vi "KGN Get actual Values.vi"(7 "scaling":dbl, 8 "Fehler (Eingang, kein Fehler)":errorcluster, 9 "Info Cluster":T1, 10 "VISA-Referenz (Eingang)":refnum<visa-resource-name>, 11 "device (Eingang)":u32) -> (0 "Fehler (Ausgang)":errorcluster, 1 "Info Cluster out":T1, 2 "VISA-Referenz (Ausgang)":refnum<visa-resource-name>, 3 "dup device (Ausgang)":u32, 4 "actual Values Cluster":T6 {"Cluster"."PumpModeGeneral-Cluster"."dry mode" items=["wet", "dry"]; "Cluster"."PumpModeGeneral-Cluster"."control mode" items=["static", "pid"]; "Cluster"."PumpMode-Cluster"."concentratio mode" items=["water", "reagent"]; "Cluster"."PumpMode-Cluster"."Reagent" items=["HCl", "HF", "NH3", "HG", "PPM", "ORGANIC"]}, 5 "Kommandos gesendet":string, 6 "connected":bool)   [LabVIEW 2020, in "Linearisierung v2.lvlib" / "Gasteiler.lvlib" / "HovaCAL_Interface.lvlib" / "KGN.lvlib" / "KGN GUI Get.lvlib"]
uses:
  KGN GUI Get.lvlib
  Controls/Info Cluster.ctl
  Controls/Pump Dry Mode.ctl
  Controls/Pump Control Mode.ctl
  Controls/Pump Concentration Mode.ctl
  Controls/Reagent.ctl
  Controls/Controls.lvlib
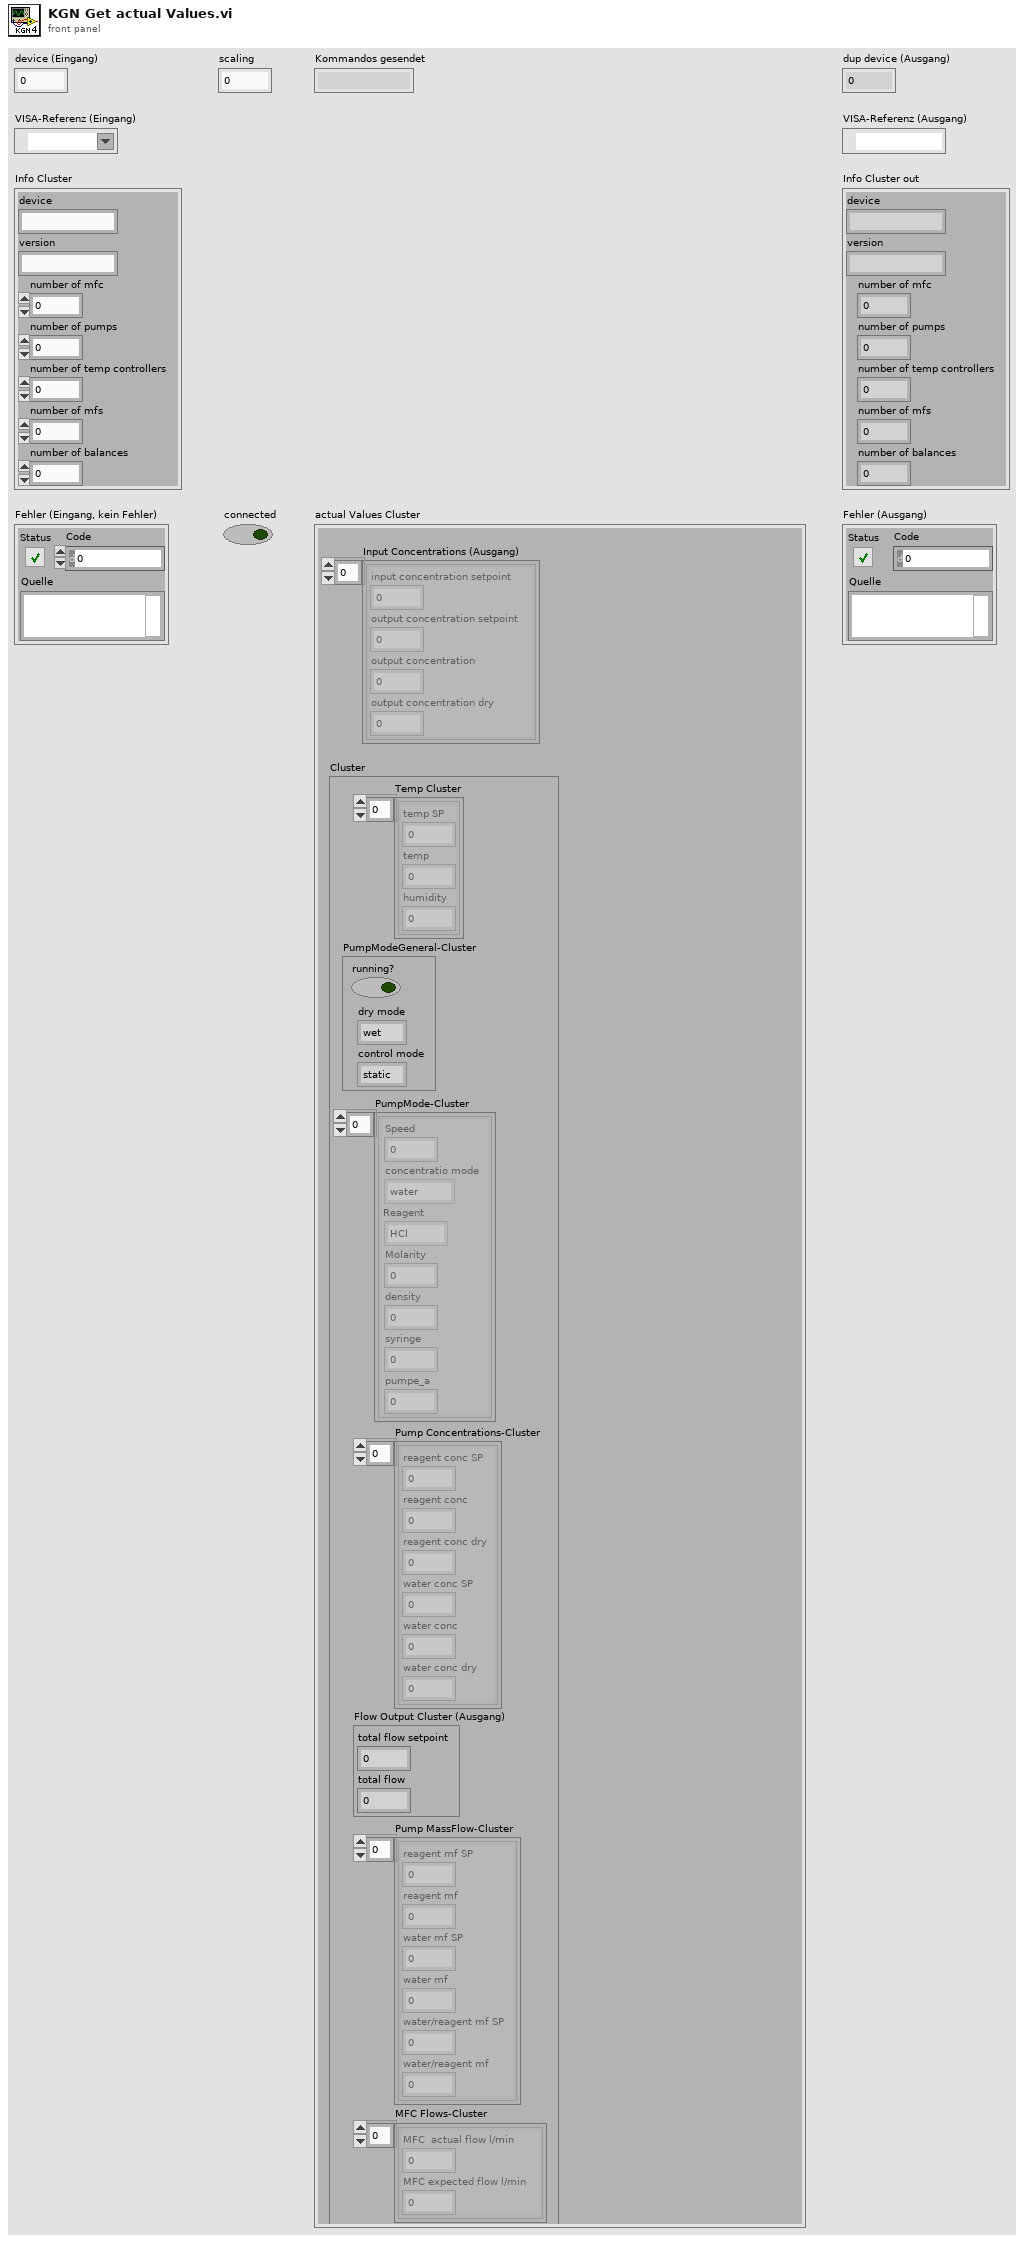
[diagram p1: front panel]
types:
  T1 = typedef "Linearisierung v2.lvlib/Gasteiler.lvlib/HovaCAL_Interface.lvlib/Controls.lvlib/Info Cluster.ctl" = cluster{"device":string, "version":string, "number of mfc":i32, "number of pumps":i32, "number of temp controllers":i32, "number of mfs":i32, "number of balances":i32}
  T2 = typedef "Linearisierung v2.lvlib/Gasteiler.lvlib/HovaCAL_Interface.lvlib/Controls.lvlib/Pump Dry Mode.ctl" = i32
  T3 = typedef "Linearisierung v2.lvlib/Gasteiler.lvlib/HovaCAL_Interface.lvlib/Controls.lvlib/Pump Control Mode.ctl" = u32
  T4 = typedef "Linearisierung v2.lvlib/Gasteiler.lvlib/HovaCAL_Interface.lvlib/Controls.lvlib/Pump Concentration Mode.ctl" = i32
  T5 = typedef "Linearisierung v2.lvlib/Gasteiler.lvlib/HovaCAL_Interface.lvlib/Controls.lvlib/Reagent.ctl" = i32
  T6 = cluster{"Input Concentrations (Ausgang)":cluster{"input concentration setpoint":dbl, "output concentration setpoint":dbl, "output concentration":dbl, "output concentration dry":dbl}[], "Cluster":cluster{"Temp Cluster":cluster{"temp SP":dbl, "temp":dbl, "humidity":dbl}[], "PumpModeGeneral-Cluster":cluster{"running?":bool, "dry mode":T2, "control mode":T3}, "PumpMode-Cluster":cluster{"Speed":dbl, "concentratio mode":T4, "Reagent":T5, "Molarity":dbl, "density":dbl, "syringe":dbl, "pumpe_a":dbl}[], "Pump Concentrations-Cluster":cluster{"reagent conc SP":dbl, "reagent conc":dbl, "reagent conc dry":dbl, "water conc SP":dbl, "water conc":dbl, "water conc dry":dbl}[], "Flow Output Cluster (Ausgang)":cluster{"total flow setpoint":dbl, "total flow":dbl}, "Pump MassFlow-Cluster":cluster{"reagent mf SP":dbl, "reagent mf":dbl, "water mf SP":dbl, "water mf":dbl, "water/reagent mf SP":dbl, "water/reagent mf":dbl}[], "MFC Flows-Cluster":cluster{"MFC  actual flow l/min":dbl, "MFC expected flow l/min":dbl}[]}}
  T7 = cluster{"input concentration setpoint":dbl, "output concentration setpoint":dbl, "output concentration":dbl, "output concentration dry":dbl}[]
  T8 = cluster{"temp SP":dbl, "temp":dbl, "humidity":dbl}[]
  T9 = cluster{"running?":bool, "dry mode":T2, "control mode":T3}
  T10 = cluster{"Speed":dbl, "concentratio mode":T4, "Reagent":T5, "Molarity":dbl, "density":dbl, "syringe":dbl, "pump_a":dbl}[]
  T11 = cluster{"reagent conc SP":dbl, "reagent conc":dbl, "reagent conc dry":dbl, "water conc SP":dbl, "water conc":dbl, "water conc dry":dbl}[]
  T12 = cluster{"reagent mf SP":dbl, "reagent mf":dbl, "water mf SP":dbl, "water mf":dbl, "water/reagent mf SP":dbl, "water/reagent mf":dbl}[]
  T13 = cluster{"total flow setpoint":dbl, "total flow":dbl}
  T14 = cluster{"MFC  actual flow l/min":dbl, "MFC expected flow l/min":dbl}[]
  T15 = cluster{"Temp Cluster":cluster{"temp SP":dbl, "temp":dbl, "humidity":dbl}[], "PumpModeGeneral-Cluster":cluster{"running?":bool, "dry mode":T2, "control mode":T3}, "PumpMode-Cluster":cluster{"Speed":dbl, "concentratio mode":T4, "Reagent":T5, "Molarity":dbl, "density":dbl, "syringe":dbl, "pump_a":dbl}[], "Pump Concentrations-Cluster":cluster{"reagent conc SP":dbl, "reagent conc":dbl, "reagent conc dry":dbl, "water conc SP":dbl, "water conc":dbl, "water conc dry":dbl}[], "Flow Output Cluster (Ausgang)":cluster{"total flow setpoint":dbl, "total flow":dbl}, "Pump MassFlow-Cluster":cluster{"reagent mf SP":dbl, "reagent mf":dbl, "water mf SP":dbl, "water mf":dbl, "water/reagent mf SP":dbl, "water/reagent mf":dbl}[], "MFC Flows (Ausgang)":cluster{"MFC  actual flow l/min":dbl, "MFC expected flow l/min":dbl}[]}
  T16 = cluster{"Input Concentrations (Ausgang)":cluster{"input concentration setpoint":dbl, "output concentration setpoint":dbl, "output concentration":dbl, "output concentration dry":dbl}[], cluster{"Temp Cluster":cluster{"temp SP":dbl, "temp":dbl, "humidity":dbl}[], "PumpModeGeneral-Cluster":cluster{"running?":bool, "dry mode":T2, "control mode":T3}, "PumpMode-Cluster":cluster{"Speed":dbl, "concentratio mode":T4, "Reagent":T5, "Molarity":dbl, "density":dbl, "syringe":dbl, "pump_a":dbl}[], "Pump Concentrations-Cluster":cluster{"reagent conc SP":dbl, "reagent conc":dbl, "reagent conc dry":dbl, "water conc SP":dbl, "water conc":dbl, "water conc dry":dbl}[], "Flow Output Cluster (Ausgang)":cluster{"total flow setpoint":dbl, "total flow":dbl}, "Pump MassFlow-Cluster":cluster{"reagent mf SP":dbl, "reagent mf":dbl, "water mf SP":dbl, "water mf":dbl, "water/reagent mf SP":dbl, "water/reagent mf":dbl}[], "MFC Flows (Ausgang)":cluster{"MFC  actual flow l/min":dbl, "MFC expected flow l/min":dbl}[]}}
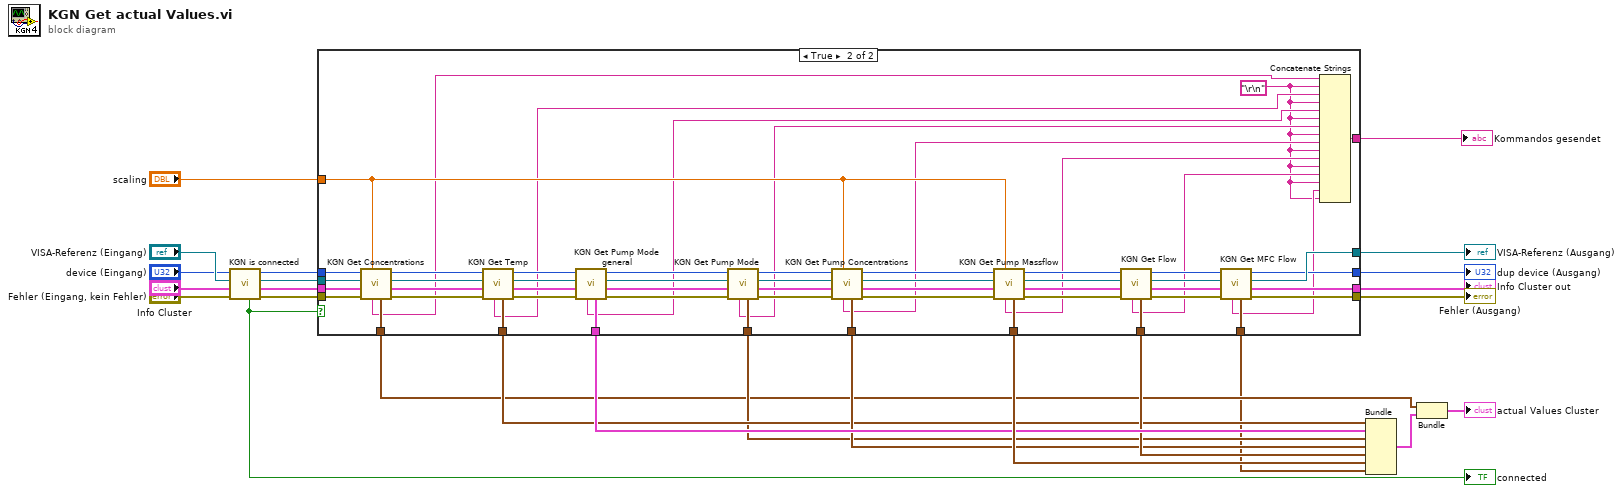
[diagram p0: block diagram]
diagram:
  n1 = call "KGN is connected.vi"("VISA-Ressourcenname"="VISA-Referenz (Eingang)", "device"="device (Eingang)") -> ("VISA-Ressourcenname out"=w22:refnum<visa-resource-name>, "dup device out"=w21:u32, "Boolesch"=w20:bool)  [unwired: 6 in, 1 out]
  "connected" <- w20
  n2 = case shown="True" w20 {
    tunnel: "Fehler (Eingang, kein Fehler)" -> [w27 w82]
    tunnel: [w27 w39] -> w8
    tunnel: w21 -> [w26 w81]
    tunnel: [_ w66] -> w6
    tunnel: "Info Cluster" -> [w24 w68]
    tunnel: [w26 w43] -> w9
    tunnel: "scaling" -> [_ w50]
    tunnel: [_ w57] -> w11
    tunnel: [_ w63] -> w12
    tunnel: [_ w54] -> w13
    tunnel: [_ w49] -> w14
    tunnel: [_ w60] -> w15
    tunnel: [_ w53] -> w18
    tunnel: w22 -> [w25 w67]
    tunnel: [w25 w45] -> w23
    tunnel: [w24 w41] -> w3
    tunnel: [_ w38] -> w2
    tunnel: [_ w28] -> w1
    frame False {
    }
    frame True {
      w29 = "\r\n"
      n3 = call "KGN Get Concentrations.vi"("scaling"=w50, "Fehler (Eingang, kein Fehler)"=w82, "Info Cluster"=w68, "VISA-Ressourcenname"=w67, "device (Eingang)"=w81) -> ("Fehler (Ausgang)"=w80:errorcluster, "Info Cluster out"=w65:T1, "VISA-Ressourcenname out"=w64:refnum<visa-resource-name>, "dup device (Ausgang)"=w79:u32, "Input Concentrations (Ausgang)"=w66:T7, "Kommandos gesendet"=w37:string)  [unwired: 1 in]
      n4 = call "KGN Get Temp.vi"("Fehler (Eingang, kein Fehler)"=w80, "Info Cluster"=w65, "VISA-Ressourcenname"=w64, "device (Eingang)"=w79) -> ("Fehler (Ausgang)"=w76:errorcluster, "Info Cluster out"=w61:T1, "VISA-Ressourcenname out"=w62:refnum<visa-resource-name>, "dup device (Ausgang)"=w74:u32, "Temp Cluster"=w63:T8, "Kommandos gesendet"=w36:string)  [unwired: 2 in]
      n5 = call "KGN Get Pump Mode general.vi"("Fehler (Eingang, kein Fehler)"=w76, "Info Cluster"=w61, "VISA-Ressourcenname"=w62, "device (Eingang)"=w74) -> ("Fehler (Ausgang)"=w75:errorcluster, "Info Cluster out"=w59:T1, "VISA-Ressourcenname out"=w58:refnum<visa-resource-name>, "dup device (Ausgang)"=w73:u32, "PumpModeGeneral-Cluster"=w60:T9, "Kommandos gesendet"=w35:string)  [unwired: 2 in]
      n6 = call "KGN Get Pump Mode.vi"("Fehler (Eingang, kein Fehler)"=w75, "Info Cluster"=w59, "VISA-Ressourcenname"=w58, "device (Eingang)"=w73) -> ("Fehler (Ausgang)"=w77:errorcluster, "Info Cluster out"=w56:T1, "VISA-Ressourcenname out"=w55:refnum<visa-resource-name>, "dup device (Ausgang)"=w78:u32, "PumpMode-Cluster"=w57:T10, "Kommandos gesendet"=w34:string)  [unwired: 2 in]
      n7 = call "KGN Get Pump Concentrations.vi"("scaling"=w50, "Fehler (Eingang, kein Fehler)"=w77, "Info Cluster"=w56, "VISA-Ressourcenname"=w55, "device (Eingang)"=w78) -> ("Fehler (Ausgang)"=w71:errorcluster, "Info Cluster out"=w52:T1, "VISA-Ressourcenname out"=w51:refnum<visa-resource-name>, "dup device (Ausgang)"=w72:u32, "Pump Concentrations-Cluster"=w54:T11, "Kommandos gesendet"=w33:string)  [unwired: 1 in]
      n8 = call "KGN Get Pump Massflow.vi"("scaling"=w50, "Fehler (Eingang, kein Fehler)"=w71, "Info Cluster"=w52, "VISA-Referenz (Eingang)"=w51, "device (Eingang)"=w72) -> ("Fehler (Ausgang)"=w69:errorcluster, "Info Cluster out"=w47:T1, "VISA-Referenz (Ausgang)"=w48:refnum<visa-resource-name>, "dup device (Ausgang)"=w70:u32, "Pump MassFlow-Cluster"=w53:T12, "Kommandos gesendet"=w32:string)  [unwired: 1 in]
      n9 = call "KGN Get Flow.vi"("Fehler (Eingang, kein Fehler)"=w69, "Info Cluster"=w47, "VISA-Referenz (Eingang)"=w48, "device (Eingang)"=w70) -> ("Fehler (Ausgang)"=w40:errorcluster, "Info Cluster out"=w42:T1, "VISA-Referenz (Ausgang)"=w46:refnum<visa-resource-name>, "dup device"=w44:u32, "Flow Output Cluster (Ausgang)"=w49:T13, "Kkommandos gesendet"=w31:string)  [unwired: 2 in]
      n10 = call "KGN Get MFC Flow.vi"("Fehler (Eingang, kein Fehler)"=w40, "Info Cluster"=w42, "VISA-Ressourcenname"=w46, "device (Eingang)"=w44) -> ("Fehler (Ausgang)"=w39:errorcluster, "Info Cluster out"=w41:T1, "VISA-Ressourcenname out"=w45:refnum<visa-resource-name>, "dup device (Ausgang)"=w43:u32, "MFC Flows (Ausgang)"=w38:T14, "Kommandos gesendet"=w30:string)  [unwired: 2 in]
      n11 = Concatenate Strings(w37, w29, w36, w29, w35, w29, w34, w29, w33, w29, w32, w29, w31, w29, w30, w29) -> (w28:string)
    }
  }
  "VISA-Referenz (Ausgang)" <- w23
  "dup device (Ausgang)" <- w9
  "Fehler (Ausgang)" <- w8
  "Info Cluster out" <- w3
  "Kommandos gesendet" <- w1
  n12 = Bundle("Temp Cluster"=w12, "PumpModeGeneral-Cluster"=w15, "PumpMode-Cluster"=w11, "Pump Concentrations-Cluster"=w13, "Flow Output Cluster (Ausgang)"=w14, "Pump MassFlow-Cluster"=w18, "MFC Flows (Ausgang)"=w2) -> (w5:T15)  [unwired: 1 in]
  n13 = Bundle("Input Concentrations (Ausgang)"=w6, w5) -> (→"actual Values Cluster":T16)  [unwired: 1 in]
